vi "Open_Instr.vi"(8 "error in (no error)":errorcluster caption="entrée d'erreur (pas d'erreur)", 11 "Class Multimeter Power_Supply en entrée":refnum<class "Class Instrument Power_Supply.lvclass">) -> (0 "error out":errorcluster caption="sortie d'erreur", 3 "Class Multimeter Power_Supply en sortie":refnum<class "Class Instrument Power_Supply.lvclass">)   [LabVIEW 2020, in "Library Instrument & Equipement.lvlib" / "Library Instruments.lvlib" / "Class Instrument Power_Supply.lvclass"]
uses:
  Class Instrument Power_Supply.lvclass
  Class Instrument Power_Supply.lvclass/Class Instrument Power_Supply.ctl
  Instrument (Default)/Class Instrument (Default).lvclass
  Power_Supply/Power_Supply (Default)/Power_Supply (Default).lvclass
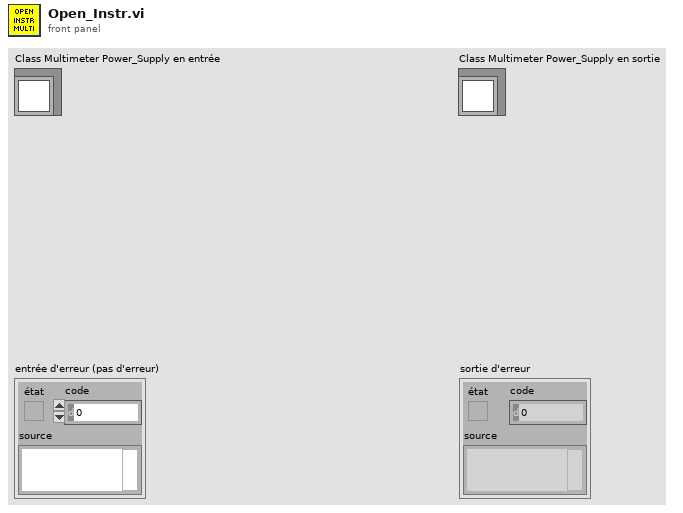
[diagram p1: front panel]
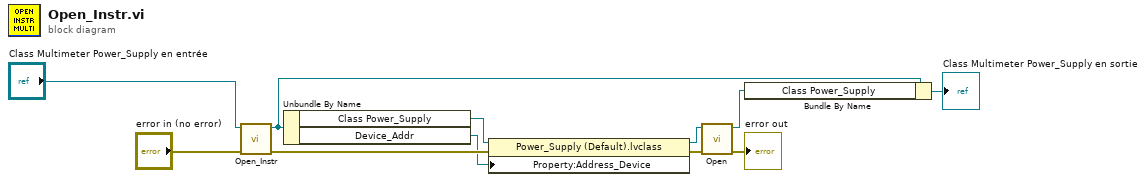
[diagram p0: block diagram]
diagram:
  n1 = call-parent "Open_Instr.vi"("error in (no error)"="error in (no error)", "Class Multimeter (Default) en entrée"="Class Multimeter Power_Supply en entrée") -> ("error out"=w8:errorcluster, "Class Multimeter (Default) en sortie"=w1:refnum<class "Class Instrument Power_Supply.lvclass">)  [unwired: 8 in]
  n2 = Unbundle By Name(w1) -> ("Class Power_Supply"=w5:refnum<class "Power_Supply (Default).lvclass">, "Device_Addr"=w6:refnum<visa-resource-name>)
  n3 = property class="Power_Supply (Default).lvclass"(reference=w5, error in=w8, "Property:Address_Device"=w6) -> (reference out=w4:refnum<class "Power_Supply (Default).lvclass">, error out=w7:errorcluster)
  n4 = call-dynamic "Open.vi"("error in (no error)"=w7, "Power_Supply (Default) en entrée"=w4) -> ("error out"=→"error out":errorcluster, "Power_Supply (Default) en sortie"=w3:refnum<class "Power_Supply (Default).lvclass">)  [unwired: 8 in]
  n5 = Bundle By Name(cluster=w1, "Class Power_Supply"=w3) -> (→"Class Multimeter Power_Supply en sortie":refnum<class "Class Instrument Power_Supply.lvclass">)
